vi "Final_State_Feedback_code.vi"() -> ()   [LabVIEW 2019]
uses:
  <vilib>/MakerHub/LINX/LMH-LINX.lvlib
  <vilib>/MakerHub/LINX/Public/Sensors/Accelerometer/MPU60X0/MPU60X0.lvlib
  <vilib>/MakerHub/LINX/Public/Sensors/Accelerometer/MPU60X0/DeviceAddresses.ctl
  <vilib>/MakerHub/LINX/Public/Sensors/Accelerometer/MPU60X0/AccelFullScaleRanges.ctl
  <vilib>/MakerHub/LINX/Public/Sensors/Accelerometer/MPU60X0/GyroFullScaleRanges.ctl
  <vilib>/MakerHub/LINX/Public/Utilities/Open Serial.vi
  <vilib>/MakerHub/LINX/Public/Peripherals/PWM/PWM Set Duty Cycle N Chans.vi
  <vilib>/MakerHub/LINX/Public/Peripherals/Digital/Digital Write N Chans.vi
panel:
  out "PWM":dbl[](graph)=[0.4072750936243316, 0.4072750936243316]
  out "Angle Reading":dbl(graph)=0.09983265430809692
  out "atan2(y,x)":dbl=0.09623213711585005
  in  "setpoint":dbl=0.15
  in  "alpha":dbl=0.98
  out "PWM":dbl[](array[numeric])=[0.4072750936243316, 0.4072750936243316]
  in  "k theta dot":dbl=-0.25
  in  "k theta":dbl=8.139999999999999
  out "Loop Rate (Hz)":u32=43
  in  "y":dbl=-377.638 format="%#_13g"
  out "angle rad":dbl=0.09983265430809692 format="%0.5f"
  in  "stop":bool
  out "Acceleration Data (g)":T1={"X Axis"=368, "Y Axis"=1404, "Z Axis"=14540}
  in  "Baud Rate Override":u32=115200
  in  "Serial Port":refnum<visa-resource-name>="COM8"
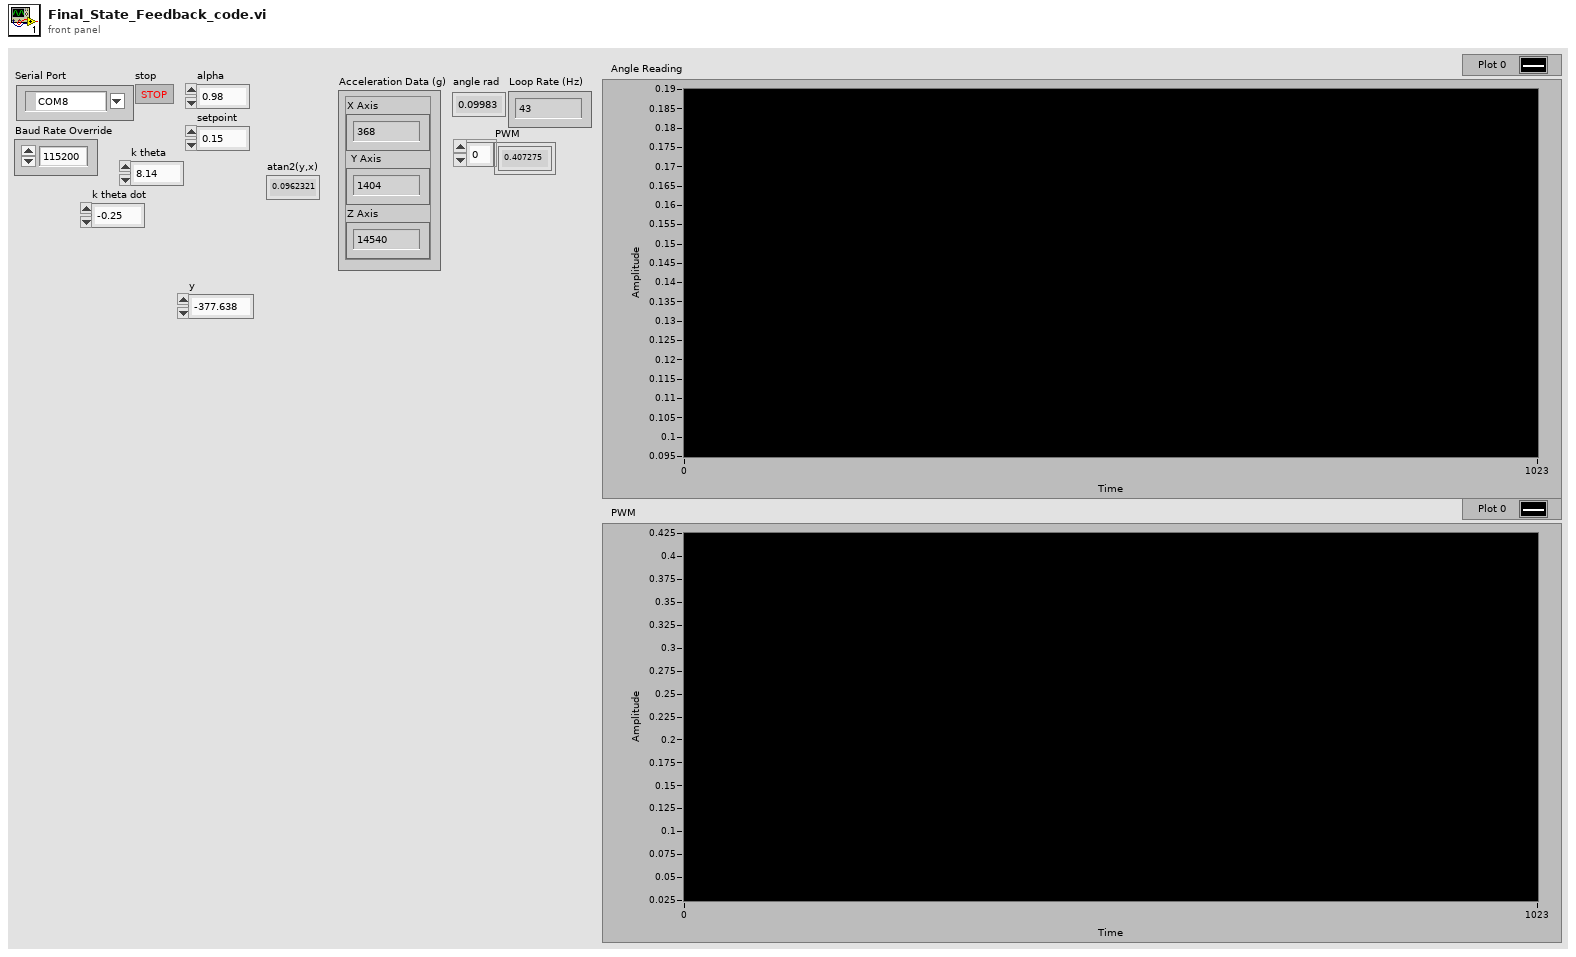
[diagram p1: front panel]
types:
  T1 = cluster{"X Axis":i16, "Y Axis":i16, "Z Axis":i16}
  T2 = typedef "LMH-LINX.lvlib/MPU60X0.lvlib/GyroFullScaleRanges.ctl" = enum8{"±250 °/s", "±500 °/s", "±1000 °/s", "±2000 °/s"}
  T3 = typedef "LMH-LINX.lvlib/MPU60X0.lvlib/AccelFullScaleRanges.ctl" = enum16{"±2g", "±4g", "±8g", "±16g"}
  T4 = typedef "LMH-LINX.lvlib/MPU60X0.lvlib/DeviceAddresses.ctl" = enum16{"0x68", "0x69"}
  T5 = typedef "LMH-LINX.lvlib/LINX Ref.ctl" = cluster{"IO":T6, "Interface":T7, "LINX Device Config":T8}
  T6 = typedef "LMH-LINX.lvlib/Platform.ctl" = enum16{"Remote", "Local"}
  T7 = typedef "LMH-LINX.lvlib/Interface.ctl" = enum16{"Serial", "TCP"}
  T8 = typedef "LMH-LINX.lvlib/Device.lvlib/LINX Device Config.ctl" = cluster{"Interface":T7, "COM Port":refnum<visa-resource-name>, "TCP Configuration":T9, "Device Family":u8, "Device ID":u8, "Device Name":string, "TCP Ref":refnum<k5>, "Channels":T10}
  T9 = typedef "LMH-LINX.lvlib/Device.lvlib/TCP Config.ctl" = cluster{"IP Address":string, "Port":u16}
  T10 = typedef "LMH-LINX.lvlib/Channels.ctl" = cluster{"DI":u8[], "DO":u8[], "AI":u8[], "AO":u8[], "PWM":u8[], "QE":u8[], "UART":u8[], "I2C 2":u8[], "SPI":u8[], "CAN":u8[], "Servo":u8[], "AI Ref (V)":dbl, "AI Resolution (Bits)":u8, "AO Ref (V)":dbl, "AO Resolution (Bits)":u8}
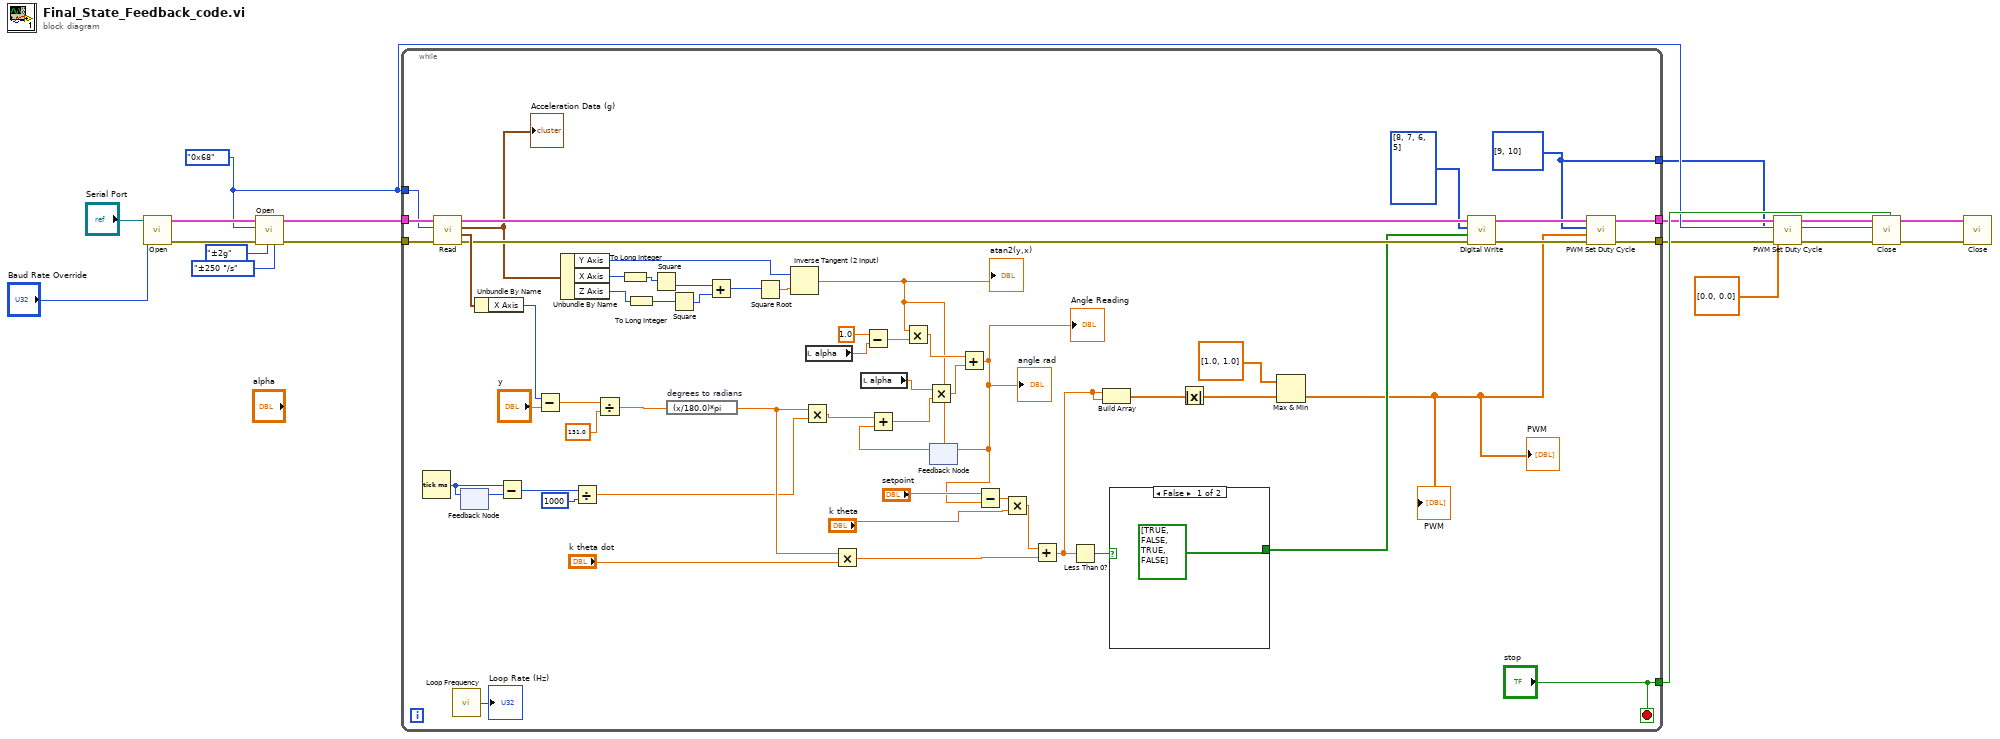
[diagram p0: block diagram]
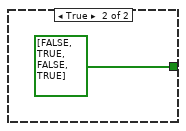
[diagram p2: hidden frame]
diagram:
  w7 = DeviceAddresses."0x68" ("I2C Slave Address")
  n1 = call-poly <vilib>:"Open.vi"("Baud Rate Override"="Baud Rate Override", "Serial Port"="Serial Port") -> ("Error Out"=w13:errorcluster, "LINX Resource"=w18:T5)  [unwired: 7 in, 1 out]
  n2 = call <vilib>:"Open.vi"("Gyro Full Scale Range"=GyroFullScaleRanges."±250 °/s", "Accel Full Scale Range"=AccelFullScaleRanges."±2g", "Error In"=w13, "I2C Slave Address"=w7, "LINX Resource"=w18) -> ("Error Out"=w14:errorcluster, "LINX Resource Out"=w17:T5)  [unwired: 5 in]
  n3 = while {
    tunnel: w17 -> [w77]
    tunnel: [w63] -> w6
    tunnel: [w62] -> w5
    tunnel: w14 -> [w76]
    tunnel: w7 -> [w75]
    tunnel: ["stop"] -> w8
    tunnel: [w21] -> w2
    stop <- "stop" stop-if-true
    w21 = u8[] [9, 10] ("PWM Channels")
    n4 = Tick Count (ms)() -> (millisecond timer value=w70:u32)
    n5 = call <vilib>:"Read.vi"("Error In"=w76, "I2C Slave Address"=w75, "LINX Resource"=w77) -> ("Error Out"=w60:errorcluster, "Gyro  Data (dps)"=w74:T1, "Acceleration Data (g)"=w48:T1, "LINX Resource Out"=w65:T5)  [unwired: 4 in, 1 out]
    "Acceleration Data (g)" <- w48
    n6 = call <vilib>:"Loop Frequency.vi"() -> ("Loop Rate (Hz)"=→"Loop Rate (Hz)":u32)
    n7 = feedback-in #1(w70) -> ()
    n8 = feedback #1() -> (w69:u32)  [unwired: 1 in]
    n9 = Unbundle By Name(w74) -> ("X Axis"=w58:i16)
    n10 = Subtract(x=w70, y=w69) -> (x-y=w68:u32)
    n11 = Subtract(x=w58, y="y") -> (x-y=w72:dbl)
    n12 = Unbundle By Name(w48) -> ("Y Axis"=w36:i16, "X Axis"=w35:i16, "Z Axis"=w34:i16)
    n13 = Divide(x=w68, y=u32 1000) -> (x/y=w26:dbl)
    n14 = Divide(x=w72, y=131.0) -> (x/y=w49:dbl)
    n15 = To Long Integer(number=w35) -> (32bit integer=w29:i32)
    n16 = To Long Integer(number=w34) -> (32bit integer=w28:i32)
    n17 = Square(x=w29) -> (x^2=w33:i32)
    n18 = expression code="(x/180.0)*pi" "degrees to radians"(w49) -> (w27:dbl)
    n19 = Square(x=w28) -> (x^2=w32:i32)
    n20 = Add(x=w33, y=w32) -> (x+y=w31:i32)
    n21 = Square Root(x=w31) -> (sqrt(x)=w30:dbl)
    n22 = Inverse Tangent (2 Input)(1:w30, 2:w36) -> (0:w25:dbl)
    "atan2(y,x)" <- w25
    n23 = Multiply(x=w27, y=w26) -> (x*y=w24:dbl)
    n24 = local read "alpha"() -> (w46:dbl)
    n25 = Multiply(x=w27, y="k theta dot") -> (x*y=w38:dbl)
    n26 = local read "alpha"() -> (w44:dbl)
    n27 = Subtract(x=1.0, y=w46) -> (x-y=w45:dbl)
    n28 = Multiply(x=w25, y=w45) -> (x*y=w43:dbl)
    n29 = feedback #2(w25) -> (w23:dbl)
    n30 = Add(x=w24, y=w23) -> (x+y=w22:dbl)
    n31 = Multiply(x=w44, y=w22) -> (x*y=w42:dbl)
    n32 = Add(x=w43, y=w42) -> (x+y=w20:dbl)
    "angle rad" <- w20
    "Angle Reading" <- w20
    n33 = feedback-in #2(w20) -> ()
    n34 = Subtract(x="setpoint", y=w20) -> (x-y=w40:dbl)
    n35 = Multiply(x=w40, y="k theta") -> (x*y=w56:dbl)
    n36 = Add(x=w56, y=w38) -> (x+y=w53:dbl)
    n37 = Less Than 0?(x=w53) -> (x < 0?=w55:bool)
    n38 = Build Array(w53, w53) -> (w52:dbl[])
    n39 = case shown="False" w55 {
      tunnel: [bool[] [TRUE, FALSE, TRUE, FALSE] ("Values") bool[] [FALSE, TRUE, FALSE, TRUE] ("Values")] -> w54
      frame False {
      }
      frame True {
      }
    }
    n40 = Absolute Value(x=w52) -> (abs(x)=w51:dbl[])
    n41 = Max & Min(x=dbl[] [1.0, 1.0], y=w51) -> (min(x,y)=w19:dbl[])  [unwired: 1 out]
    "PWM" <- w19
    "PWM" <- w19
    n42 = call-poly <vilib>:"Digital Write.vi"("Error In"=w60, "Values"=w54, "DO Channels"=u8[] [8, 7, 6, 5], "LINX Resource"=w65) -> ("Error Out"=w61:errorcluster, "LINX Resource Out"=w64:T5)  [unwired: 6 in]
    n43 = call-poly <vilib>:"PWM Set Duty Cycle.vi"("Error In"=w61, "Duty Cycles"=w19, "PWM Channels"=w21, "LINX Resource"=w64) -> ("Error Out"=w62:errorcluster, "LINX Resource Out"=w63:T5)  [unwired: 6 in]
  }
  n44 = call-poly <vilib>:"PWM Set Duty Cycle.vi"("Error In"=w5, "Duty Cycles"=dbl[] [0.0, 0.0], "PWM Channels"=w2, "LINX Resource"=w6) -> ("Error Out"=w3:errorcluster, "LINX Resource Out"=w4:T5)  [unwired: 6 in]
  n45 = call <vilib>:"Close.vi"("Close I2C Master?"=w8, "Error In"=w3, "I2C Slave Address (0)"=w7, "LINX Resource"=w4) -> ("Error Out"=w15:errorcluster, "LINX Resource out"=w16:T5)  [unwired: 6 in]
  n46 = call <vilib>:"Close.vi"("Error In"=w15, "LINX Resource"=w16) -> ()  [unwired: 9 in, 1 out]
